vi "Result_Test.vi"(8 "error in (no error)":errorcluster caption="entrée d'erreur (pas d'erreur)", 11 "Delay en entrée":refnum<class "P2056_ExtractLog.lvclass">) -> (0 "error out":errorcluster caption="sortie d'erreur", 3 "Delay en sortie":refnum<class "P2056_ExtractLog.lvclass">)   [LabVIEW 2020, in "Library Test.lvlib" / "P2056_ExtractLog.lvclass"]
uses:
  P2056_ExtractLog.lvclass
  C:/Users/ngarcin/OneDrive - Altyor/Standard TB/Class/Test/Test (Default)/Test (Default).lvclass
  Test_Without_Instr/Test_Without_Inst.lvclass
  P2056_ExtractLog.lvclass/P2056_ExtractLog.ctl
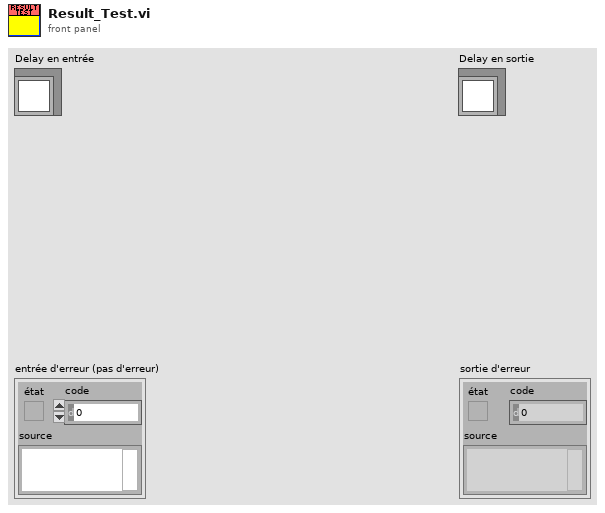
[diagram p1: front panel]
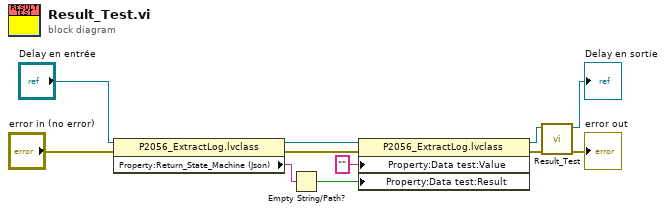
[diagram p0: block diagram]
diagram:
  n1 = property class="P2056_ExtractLog.lvclass"(reference="Delay en entrée", error in="error in (no error)") -> (reference out=w9:refnum<class "P2056_ExtractLog.lvclass">, error out=w8:errorcluster, "Property:Return_State_Machine (Json)"=w3:string)
  n2 = Empty String/Path?(string/path=w3) -> (empty?=w1:bool)
  n3 = property class="P2056_ExtractLog.lvclass"(reference=w9, error in=w8, "Property:Data test:Value"="" ("Value"), "Property:Data test:Result"=w1) -> (reference out=w5:refnum<class "P2056_ExtractLog.lvclass">, error out=w6:errorcluster)
  n4 = call-parent "Result_Test.vi"("error in (no error)"=w6, "Test_Without_Inst en entrée"=w5) -> ("error out"=→"error out":errorcluster, "Test_Without_Inst en sortie"=→"Delay en sortie":refnum<class "P2056_ExtractLog.lvclass">)  [unwired: 8 in]
